vi "Configure Limit Line Multiple Points.vi"(5 "Connected Values List":bool[](array[boolean])=[FALSE, FALSE, FALSE, FALSE, FALSE, FALSE], 6 "Amplitude Values List":dbl[](array[numeric])=[0.0, 0.0, 0.0, 0.0, 0.0, 0.0], 7 "Frequency Values List":dbl[](array[numeric])=[2000000.0, 2000000.0, 2000000.0, 2000000.0, 2000000.0, 2000000.0], 8 "error in (no error)":errorcluster, 9 "Limit Line Type (0: Upper)":i32(ring) items=["Upper", "Lower"], 10 "Limit Line Number (1: Line1)":u16(ring)=1 items=["Line1"=1, "Line2"=2], 11 "VISA resource name":refnum<visa-resource-name>) -> (0 "error out":errorcluster, 3 "VISA resource name out":refnum<visa-resource-name>)   [LabVIEW 2022 SP3, in "Agilent N934X Series.lvlib"]
doc: "Configure the limit line settings.\n\nNote:\nThis VI is only applicable for N9321C, N9322C, N9323C, N9324C models."
uses:
  <instrlib>/Agilent N934X Series/Agilent N934X Series.lvlib
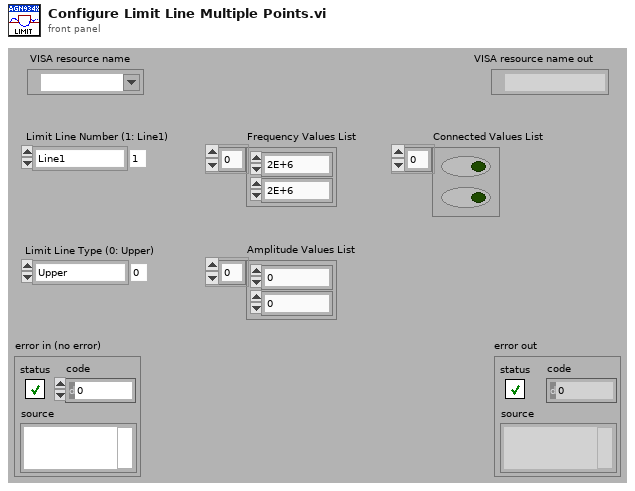
[diagram p1: front panel]
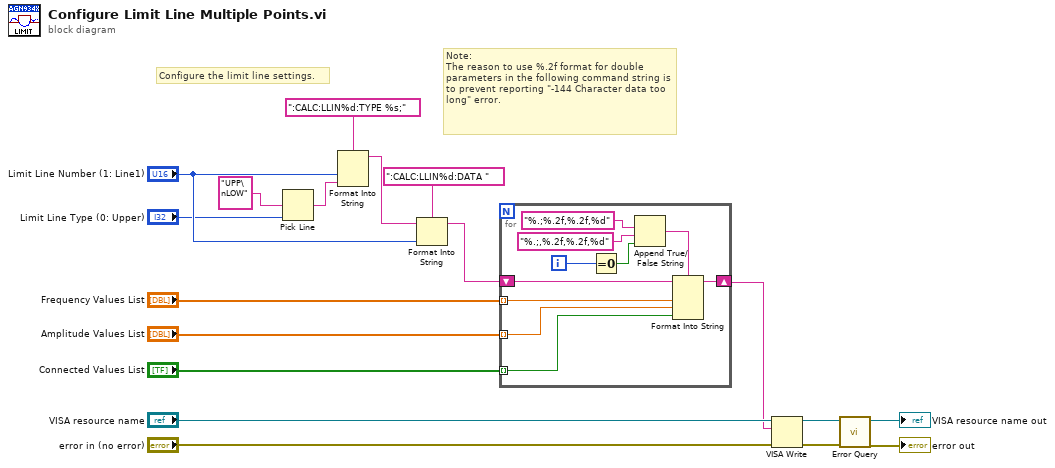
[diagram p0: block diagram]
diagram:
  # "Note: \nThe reason to use %.2f format for double parameters in the following command string is to prevent reporting \"-144 Character data too long\" error."
  # "Configure the limit line settings."
  n1 = Pick Line(multi-line string="UPP\nLOW", line index="Limit Line Type (0: Upper)") -> (output string=w7:string)  [unwired: 1 out]
  n2 = Format Into String(format string=":CALC:LLIN%d:TYPE %s;", "Limit Line Number (1: Line1)", w7) -> (resulting string=w3:string)  [unwired: 2 in, 1 out]
  n3 = Format Into String(format string=":CALC:LLIN%d:DATA ", initial string=w3, "Limit Line Number (1: Line1)") -> (resulting string=w5:string)  [unwired: 1 in, 1 out]
  n4 = for {
    shift-right: [w22] -> w1
    shift-left: w5 -> [w23]
    tunnel: "Frequency Values List" -> [w21] mode=indexing
    tunnel: "Amplitude Values List" -> [w20] mode=indexing
    tunnel: "Connected Values List" -> [w19] mode=indexing
    i -> [w24]
    n5 = Equal To 0?(x=w24) -> (x = 0?=w25:bool)
    n6 = Append True/False String(1:w25, 2:"%.;,%.2f,%.2f,%d" ("format string"), 3:"%.;%.2f,%.2f,%d" ("format string")) -> (0:w28:string)  [unwired: 1 out]
    n7 = Format Into String(format string=w28, initial string=w23, w21, w20, w19) -> (resulting string=w22:string)  [unwired: 1 in, 1 out]
  }
  n8 = VISA Write(VISA resource name="VISA resource name", write buffer=w1, error in (no error)="error in (no error)") -> (VISA resource name out=w16:refnum<visa-resource-name>, error out=w15:errorcluster)  [unwired: 1 out]
  n9 = call <instrlib>:"Error Query.vi"("error in (no error)"=w15, "VISA resource name"=w16) -> ("error out"=→"error out":errorcluster, "VISA resource name out"=→"VISA resource name out":refnum<visa-resource-name>)  [unwired: 6 in, 2 out]
